vi "Autonomous Independent.vi"() -> (3 "LED ms toggle rate":u32=500)   [LabVIEW 2013]
doc: "This VI is called when autonomous begins, and will automatically be terminated when autonomous ends. You can carry out timed or sensor driven robot movement independently without needing to return to the caller."
uses:
  Robot Global Data.vi
panel:
  out "Distance":dbl
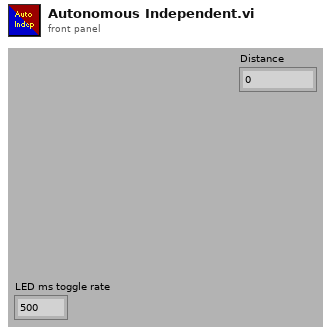
[diagram p1: front panel]
types:
  T1 = typedef "WPI_EncoderDevRef.ctl" = cluster{"DevStatus":errorcluster, "EncoderIndex":T2, "CounterIndex":T3, "DistancePerCount":dbl, "Decoding Type":T4}
  T2 = typedef "FPGA_EncoderIdx.ctl" = enum8{"Enc 0", "Enc 1", "Enc 2", "Enc 3", "Invalid"}
  T3 = typedef "FPGA_CounterCtrSystemIndex.ctl" = enum8{"Ctr 0", "Ctr 1", "Ctr 2", "Ctr 3", "Ctr 4", "Ctr 5", "Ctr 6", "Ctr 7", "Invalid"}
  T4 = typedef "WPI_EncoderType.ctl" = enum16{"1x", "2x", "4x"}
  T5 = cluster{"RightLow":dbl, "LeftLow":dbl, "RightHigh":dbl, "LeftHigh":dbl}
  T6 = typedef "WPI_MotorControlDeviceRef.ctl" = cluster{"DeviceStatus":errorcluster, "Type":enum16{"PWM", "CAN"}, "PWM":cluster{"Digital Module":T7, "PWM Channel":T8, "DeadBand":T9}, "CAN":cluster{"Device Number":u8, "Control Mode":T10, "Semaphore":T11, "Max Vout":dbl}, "Invert":bool, "TransformRef":T12, "InvTransformRef":T12}
  T7 = typedef "FPGA_TypedefDigitalModule.ctl" = enum16{"Digital Module 1", "Digital Module 2"}
  T8 = typedef "FPGA_DIOPWMChannel.ctl" = enum8{"PWM 1", "PWM 2", "PWM 3", "PWM 4", "PWM 5", "PWM 6", "PWM 7", "PWM 8", "PWM 9", "PWM 10", "Invalid"}
  T9 = typedef "WPI_PWMDeadband.ctl" = cluster{"Name":string, "maxPositivePwm":i32, "minPositivePwm":i32, "centerPwm":i32, "maxNegativePwm":i32, "minNegativePwm":i32, "angularRange":u16}
  T10 = typedef "WPI_CANJaguar_ControlMode.ctl" = enum8{"Percent VBus", "Current", "Speed", "Position", "Voltage"}
  T11 = typedef "Semaphore RefNum" = refnum<k1>
  T12 = typedef "WPI_PWMTransform_ConPane.ctl" = refnum<vi>
  T13 = typedef "WPI_ServoDeviceRef.ctl" = cluster{"DeviceStatus":errorcluster, "Digital Module":T7, "PWM Channel":T8, "DeadBand":T9}
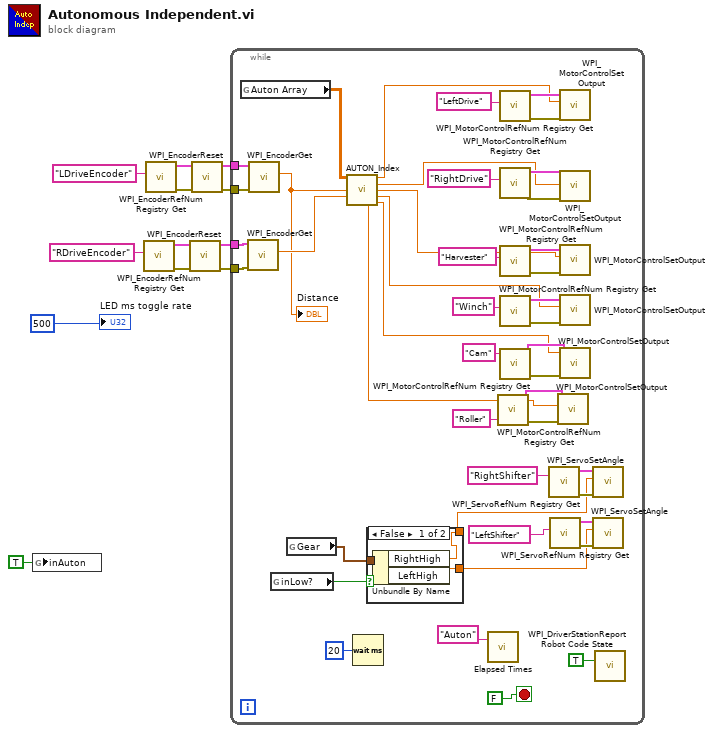
[diagram p0: block diagram]
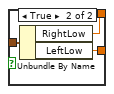
[diagram p2: hidden frame]
diagram:
  n1 = global write "Robot Global Data.vi" "inAuton"(TRUE ("inAuton")) -> ()
  n2 = call <vilib>:"WPI_EncoderRefNum Registry Get.vi"("refnum name"="RDriveEncoder") -> ("error out"=w4:errorcluster, "EncoderDevRef"=w6:T1)  [unwired: 9 in]
  n3 = call <vilib>:"WPI_EncoderRefNum Registry Get.vi"("refnum name"="LDriveEncoder") -> ("error out"=w10:errorcluster, "EncoderDevRef"=w9:T1)  [unwired: 9 in]
  n4 = call <vilib>:"WPI_EncoderReset.vi"("error in (no error)"=w4, "EncoderDevRef"=w6) -> ("error out"=w2:errorcluster, "EncoderDevRef"=w3:T1)  [unwired: 8 in]
  n5 = call <vilib>:"WPI_EncoderReset.vi"("error in (no error)"=w10, "EncoderDevRef"=w9) -> ("error out"=w7:errorcluster, "EncoderDevRef"=w8:T1)  [unwired: 8 in]
  n6 = while {
    tunnel: w8 -> [w55]
    tunnel: w7 -> [w54]
    tunnel: w3 -> [w52]
    tunnel: w2 -> [w51]
    stop <- FALSE stop-if-true
    n7 = global read "Robot Global Data.vi" "Auton Array"() -> (w29:dbl[][])
    n8 = call <vilib>:"WPI_EncoderGet.vi"("error in (no error)"=w51, "EncoderDevRef"=w52) -> ("Distance"=w50:dbl)  [unwired: 4 in, 5 out]
    n9 = call <vilib>:"WPI_EncoderGet.vi"("error in (no error)"=w54, "EncoderDevRef"=w55) -> ("Distance"=w24:dbl)  [unwired: 4 in, 5 out]
    "Distance" <- w24
    n10 = global read "Robot Global Data.vi" "inLow?"() -> (w13:bool)
    n11 = global read "Robot Global Data.vi" "Gear"() -> (w14:T5)
    n12 = call "AUTON_Index.vi"("Auton Array"=w29, "LeftEncoder"=w24, "RightEncoder"=w50) -> ("Right Drive"=w30:dbl, "Left Drive"=w31:dbl, "Harvester"=w40:dbl, "Winch"=w33:dbl, "Roller"=w25:dbl, "Cam"=w32:dbl)  [unwired: 7 in]
    n13 = Wait (ms)(milliseconds to wait=u32 20) -> ()  [unwired: 1 out]
    n14 = case shown="False" w13 {
      tunnel: [w59 w63] -> w16
      tunnel: [w58 w62] -> w15
      tunnel: w14 -> [w60 w61]
      frame False {
        n15 = Unbundle By Name(w60) -> ("RightHigh"=w59:dbl, "LeftHigh"=w58:dbl)
      }
      frame True {
        n16 = Unbundle By Name(w61) -> ("RightLow"=w63:dbl, "LeftLow"=w62:dbl)
      }
    }
    n17 = call "Elapsed Times.vi"("Call Name"="Auton") -> ()  [unwired: 2 in, 1 out]
    n18 = call <vilib>:"WPI_MotorControlRefNum Registry Get.vi"("refnum name"="Roller") -> ("error out"=w27:errorcluster, "MotorControlDevRef"=w28:T6)  [unwired: 9 in]
    n19 = call <vilib>:"WPI_MotorControlRefNum Registry Get.vi"("refnum name"="LeftDrive") -> ("error out"=w45:errorcluster, "MotorControlDevRef"=w46:T6)  [unwired: 9 in]
    n20 = call <vilib>:"WPI_MotorControlRefNum Registry Get.vi"("refnum name"="RightDrive") -> ("error out"=w41:errorcluster, "MotorControlDevRef"=w42:T6)  [unwired: 9 in]
    n21 = call <vilib>:"WPI_MotorControlRefNum Registry Get.vi"("refnum name"="Harvester") -> ("error out"=w43:errorcluster, "MotorControlDevRef"=w44:T6)  [unwired: 9 in]
    n22 = call <vilib>:"WPI_MotorControlRefNum Registry Get.vi"("refnum name"="Winch") -> ("error out"=w39:errorcluster, "MotorControlDevRef"=w35:T6)  [unwired: 9 in]
    n23 = call <vilib>:"WPI_MotorControlRefNum Registry Get.vi"("refnum name"="Cam") -> ("error out"=w36:errorcluster, "MotorControlDevRef"=w34:T6)  [unwired: 9 in]
    n24 = call <vilib>:"WPI_ServoRefNum Registry Get.vi"("refnum name"="RightShifter") -> ("error out"=w19:errorcluster, "ServoDeviceRef"=w20:T13)  [unwired: 9 in]
    n25 = call <vilib>:"WPI_ServoRefNum Registry Get.vi"("refnum name"="LeftShifter") -> ("error out"=w21:errorcluster, "ServoDeviceRef"=w22:T13)  [unwired: 9 in]
    n26 = call <vilib>:"WPI_MotorControlSetOutput.vi"("error in (no error)"=w27, "Output"=w25, "MotorControlDevRef"=w28) -> ()  [unwired: 6 in, 3 out]
    n27 = call <vilib>:"WPI_MotorControlSetOutput.vi"("error in (no error)"=w45, "Output"=w30, "MotorControlDevRef"=w46) -> ()  [unwired: 6 in, 3 out]
    n28 = call <vilib>:"WPI_MotorControlSetOutput.vi"("error in (no error)"=w41, "Output"=w31, "MotorControlDevRef"=w42) -> ()  [unwired: 6 in, 3 out]
    n29 = call <vilib>:"WPI_MotorControlSetOutput.vi"("error in (no error)"=w43, "Output"=w40, "MotorControlDevRef"=w44) -> ()  [unwired: 6 in, 3 out]
    n30 = call <vilib>:"WPI_MotorControlSetOutput.vi"("error in (no error)"=w39, "Output"=w33, "MotorControlDevRef"=w35) -> ()  [unwired: 6 in, 3 out]
    n31 = call <vilib>:"WPI_MotorControlSetOutput.vi"("error in (no error)"=w36, "Output"=w32, "MotorControlDevRef"=w34) -> ()  [unwired: 6 in, 3 out]
    n32 = call <vilib>:"WPI_ServoSetAngle.vi"("error in (no error)"=w19, "Angle"=w16, "ServoDeviceRef"=w20) -> ()  [unwired: 7 in, 2 out]
    n33 = call <vilib>:"WPI_ServoSetAngle.vi"("error in (no error)"=w21, "Angle"=w15, "ServoDeviceRef"=w22) -> ()  [unwired: 7 in, 2 out]
    n34 = call <vilib>:"WPI_DriverStationReport Robot Code State.vi"("Autonomous"=TRUE) -> ()  [unwired: 10 in, 1 out]
  }
  "LED ms toggle rate" <- u32 500 ("LED ms toggle rate")
